vi "Get Coding.vi"(10 "CoilVolt":dbl[](array[numeric])) -> (0 "Alarm":string, 1 "Distance":i32, 2 "StepE":i32, 3 "StepM":i32, 5 "Bcd":i32)   [LabVIEW 2017]
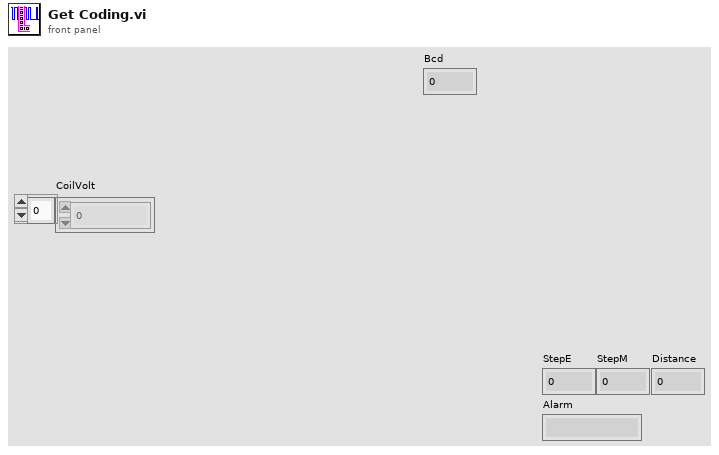
[diagram p1: front panel]
types:
  T1 = cluster{"Th_A":dbl, "Th_B":dbl, "Th_C":dbl, "ChupLimt":dbl, "ChdnLimt":dbl, "Bcd":u8, "StepMem":u32}
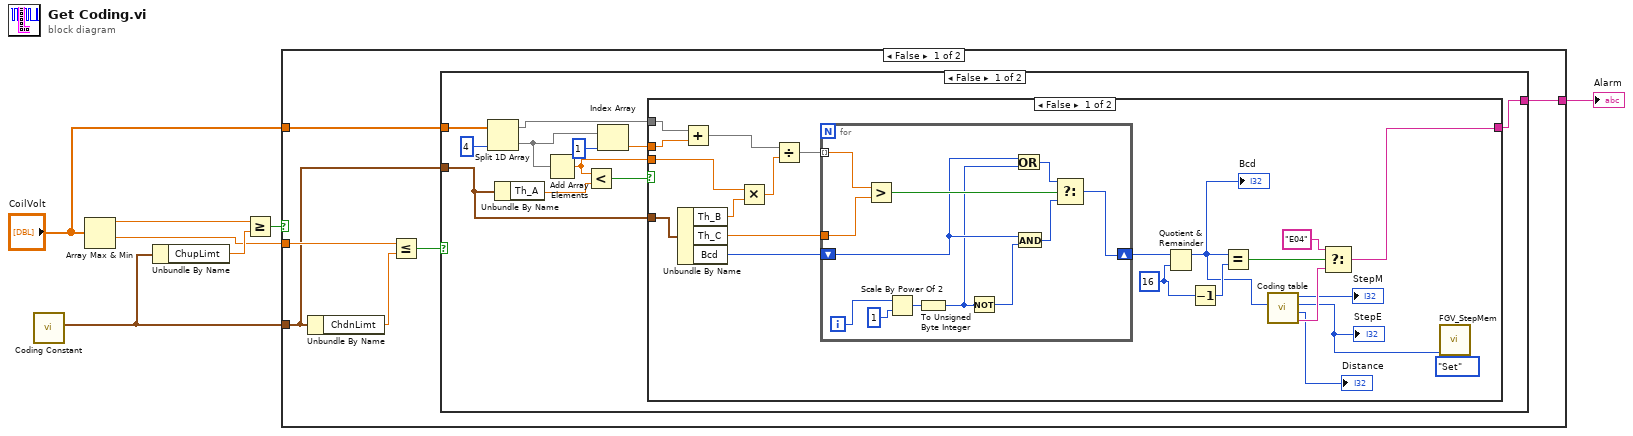
[diagram p0: block diagram]
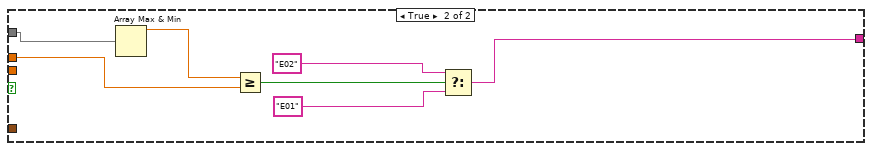
[diagram p2: hidden frame]
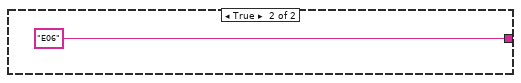
[diagram p3: hidden frame]
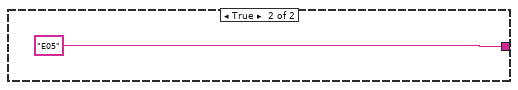
[diagram p4: hidden frame]
diagram:
  n1 = call "Coding Constant.vi"() -> ("Constant out"=w3:T1)  [unwired: 11 in]
  n2 = Array Max & Min(array="CoilVolt") -> (max value=w7:dbl, min value=w4:dbl)  [unwired: 2 out]
  n3 = Unbundle By Name(w3) -> ("ChupLimt"=w6:dbl)
  n4 = Greater Or Equal?(x=w7, y=w6) -> (x >= y?=w5:bool)
  n5 = case shown="False" w5 {
    tunnel: [w10 "E05"] -> w1
    tunnel: w4 -> [w13 _]
    tunnel: w3 -> [w9 _]
    tunnel: "CoilVolt" -> [w8 _]
    frame False {
      n6 = Unbundle By Name(w9) -> ("ChdnLimt"=w12:dbl)
      n7 = Less Or Equal?(x=w13, y=w12) -> (x <= y?=w11:bool)
      n8 = case shown="False" w11 {
        tunnel: [w19 "E06"] -> w10
        tunnel: w9 -> [w17 _]
        tunnel: w8 -> [w23 _]
        frame False {
          n9 = Split 1D Array(array=w23, index=4) -> (first subarray=w20:dbl[], second subarray=w15:dbl[])
          n10 = Unbundle By Name(w17) -> ("Th_A"=w22:dbl)
          n11 = Add Array Elements(numeric array=w15) -> (sum=w18:dbl)
          n12 = Less?(x=w18, y=w22) -> (x < y?=w21:bool)
          n13 = Index Array(array=w15, index=1) -> (element=w14:dbl)
          n14 = case shown="False" w21 {
            tunnel: w20 -> [w43 w65]
            tunnel: [w31 w60] -> w19
            tunnel: w18 -> [w46 _]
            tunnel: w17 -> [w45 _]
            tunnel: w14 -> [w42 w59]
            frame False {
              w35 = 16
              n15 = Unbundle By Name(w45) -> ("Th_B"=w44:dbl, "Th_C"=w38:dbl, "Bcd"=w37:u8)
              n16 = Add(x=w43, y=w42) -> (x+y=w40:dbl[])
              n17 = Multiply(x=w46, y=w44) -> (x*y=w41:dbl)
              n18 = Divide(x=w40, y=w41) -> (x/y=w39:dbl[])
              n19 = for {
                tunnel: w39 -> [w58] mode=indexing
                tunnel: w38 -> [w57]
                shift-right: [w52] -> w36
                shift-left: w37 -> [w55]
                i -> [w51]
                n20 = Greater?(x=w58, y=w57) -> (0:w56:bool)
                n21 = Scale By Power Of 2(n=w51, x=1) -> (x*2^n=w49:i32)
                n22 = To Unsigned Byte Integer(number=w49) -> (unsigned 8bit integer=w48:u8)
                n23 = Not(x=w48) -> (.not. x?=w47:u8)
                n24 = Or(x=w55, y=w48) -> (x .or. y?=w54:u8)
                n25 = And(x=w55, y=w47) -> (x .and. y?=w53:u8)
                n26 = Select(t=w54, s=w56, f=w53) -> (s? t:f=w52:u8)
              }
              n27 = Quotient & Remainder(x=w36, y=w35) -> (x-y*floor(x/y)=w30:i32)  [unwired: 1 out]
              "Bcd" <- w30
              n28 = Decrement(x=w35) -> (x-1=w34:i32)
              n29 = Equal?(x=w30, y=w34) -> (x = y?=w33:bool)
              n30 = call "Coding table.vi"("Bcd"=w30) -> ("Alarm"=w29:string, "Distance"=→"Distance":i32, "StepE"=w25:i32, "StepM"=→"StepM":i32)  [unwired: 7 in]
              "StepE" <- w25
              n31 = Select(t="E04", s=w33, f=w29) -> (s? t:f=w31:string)
              n32 = call "FGV_StepMem.vi"("Func"=enum16{"Set", "Get"}."Set", "StepE"=w25) -> ()  [unwired: 9 in, 1 out]
            }
            frame True {
              n33 = Array Max & Min(array=w65) -> (max value=w64:dbl)  [unwired: 3 out]
              n34 = Greater Or Equal?(x=w64, y=w59) -> (x >= y?=w63:bool)
              n35 = Select(t="E02", s=w63, f="E01") -> (s? t:f=w60:string)
            }
          }
        }
        frame True {
        }
      }
    }
    frame True {
    }
  }
  "Alarm" <- w1
